vi "Write Analyze Objects.vi"(8 "error in (no error)":errorcluster, 10 "Analyze Objects":refnum<class "Analyze BaseClass.lvclass">[](array[class]), 11 "Analyze Actor in":refnum<class "Analyze Actor.lvclass">) -> (0 "error out":errorcluster, 3 "Analyze Actor out":refnum<class "Analyze Actor.lvclass">)   [LabVIEW 2020]
uses:
  Analyze Actor.lvclass
  C:/Program Files (x86)/National Instruments/LabVIEW 2020/vi.lib/ActorFramework/Actor/Actor.lvclass
  C:/Users/AlexK/work/LabVIEW Programme/POLARIS-AS-3-Cams/Submodules/HIJ Vision/Analyze/Analyze Actor/Analyze Actor/Analyze Actor.lvclass
  Analyze Classes/Analyze BaseClass/Analyze BaseClass/Analyze BaseClass.lvclass
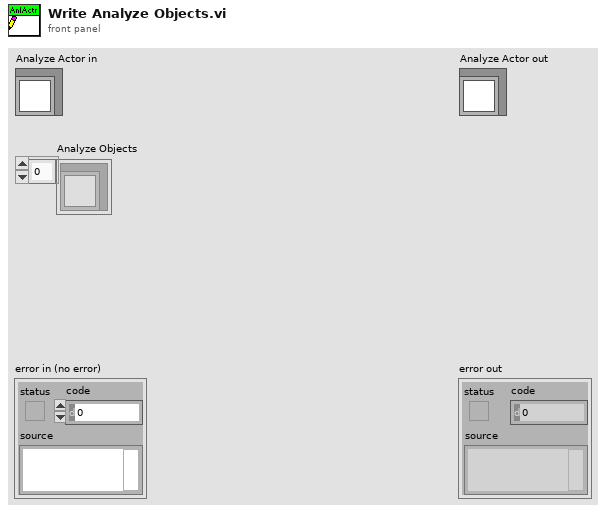
[diagram p1: front panel]
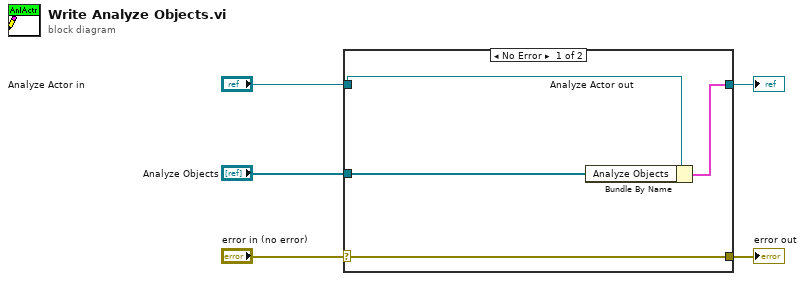
[diagram p0: block diagram]
diagram:
  n1 = case shown="No Error" "error in (no error)" {
    selector: "error in (no error)" -> [w9 w10]
    tunnel: [w9 w10] -> w4
    tunnel: [w7 w11] -> w2
    tunnel: "Analyze Actor in" -> [w8 w11]
    tunnel: "Analyze Objects" -> [w6 _]
    frame No Error {
      n2 = Bundle By Name(cluster=w8, "Analyze Objects"=w6) -> (w7:cluster{})
    }
    frame Error {
    }
  }
  "error out" <- w4
  "Analyze Actor out" <- w2
